vi "LS2A GUI MAIN.vi"() -> ()   [LabVIEW 2015]
panel:
  out "Wired":bool
  out "refnum out":refnum<file>
  out "read buffer":string
  in  "Tab Control":enum32{"Page 1", "Page 2"}(tab)
  out "Bytes Downloaded":dbl
  out "Connection Type":string
  out "Metadata 1":string
  out "Metadata 2":string
  out "Metadata 3":string
  in  "Connect to Unit":bool
  out "System Status":string
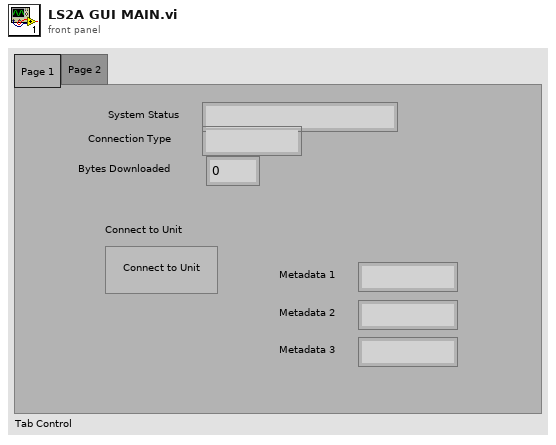
[diagram p1: front panel]
types:
  T1 = enum16{"open", "replace", "create", "open or create", "replace or create", "replace or create with confirmation"}
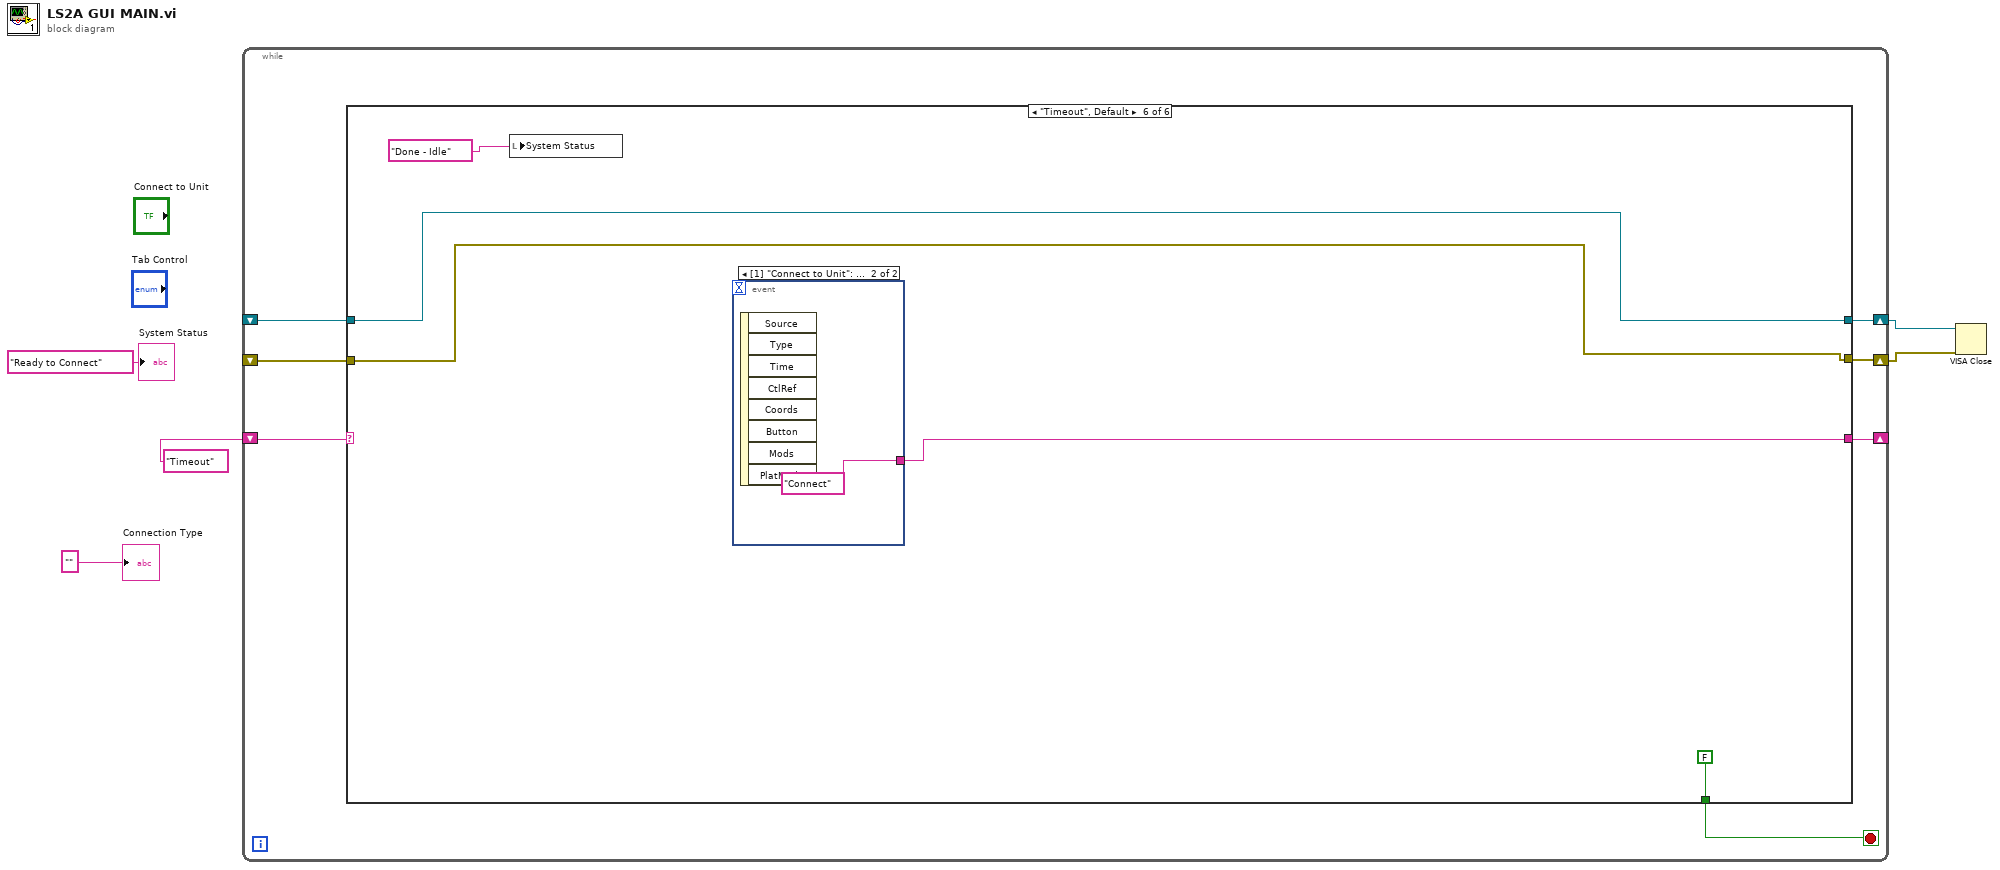
[diagram p0: block diagram]
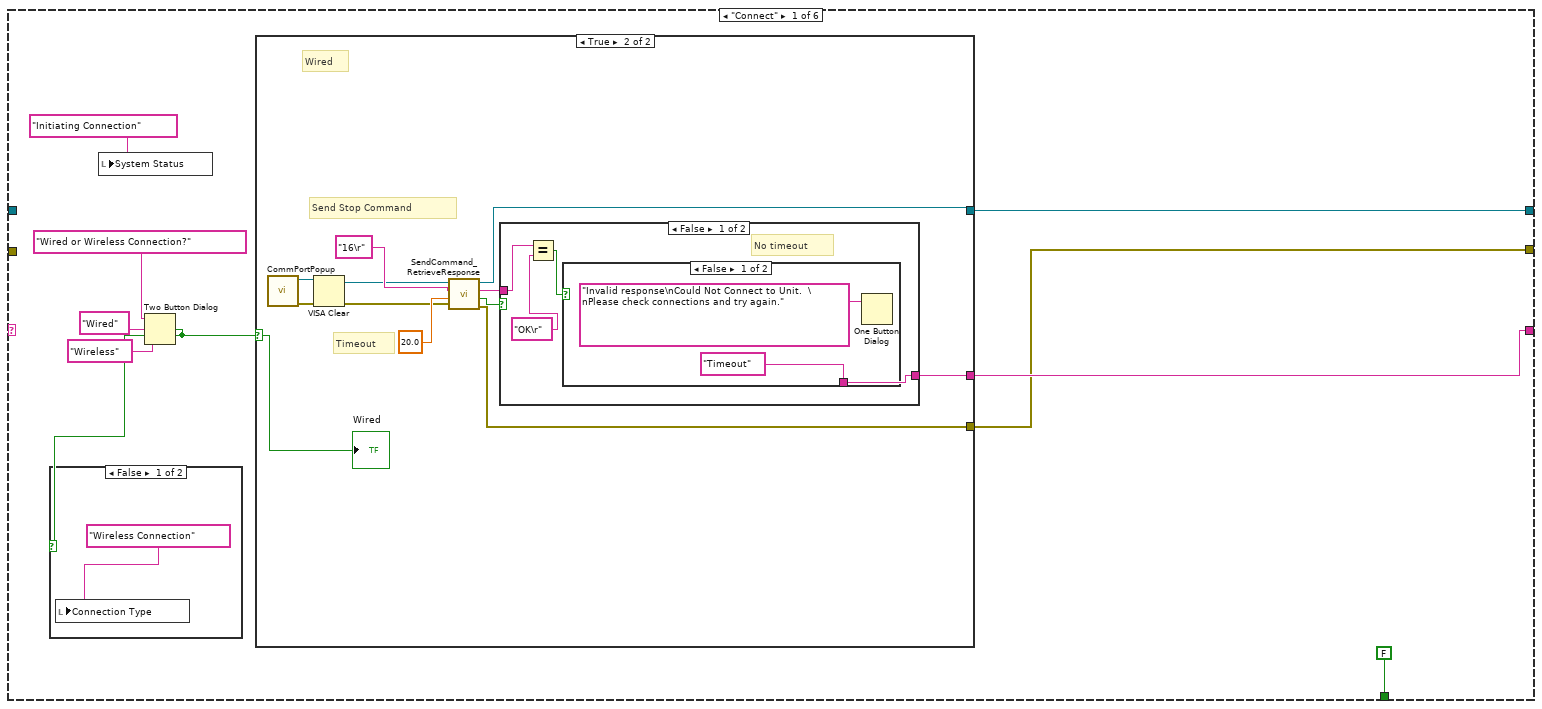
[diagram p2: hidden frame]
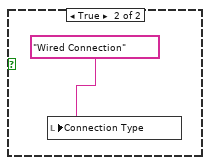
[diagram p3: hidden frame]
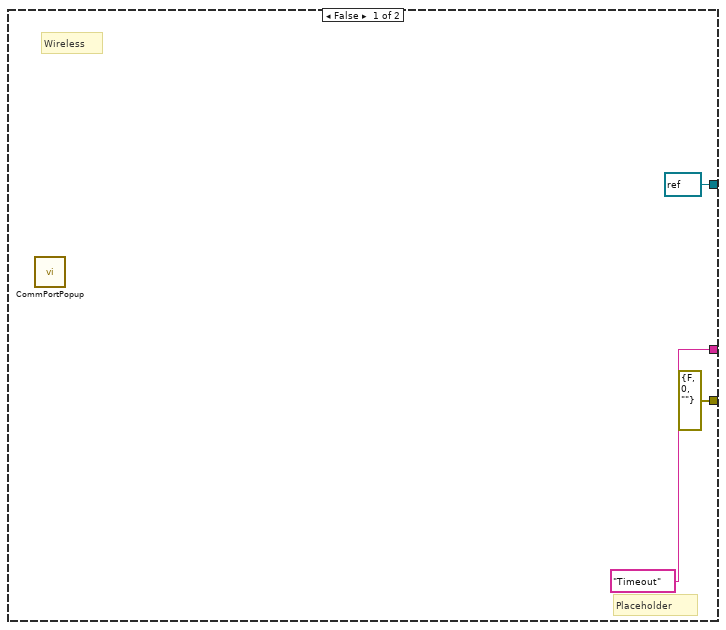
[diagram p4: hidden frame]
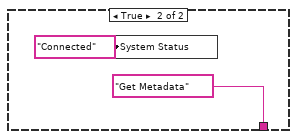
[diagram p5: hidden frame]
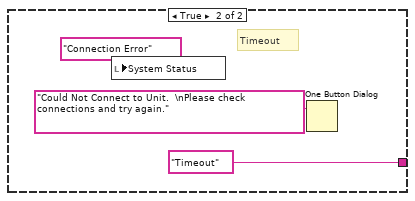
[diagram p6: hidden frame]
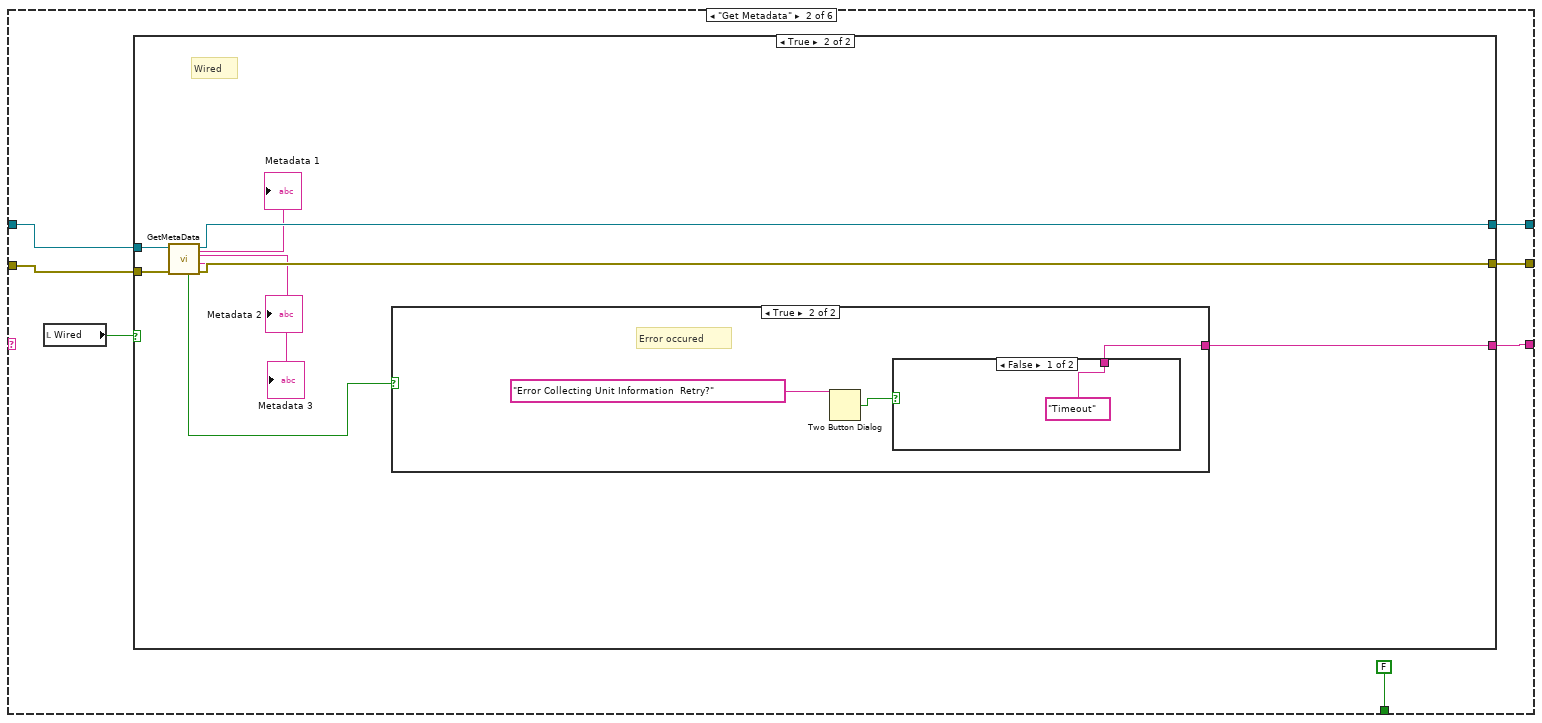
[diagram p7: hidden frame]
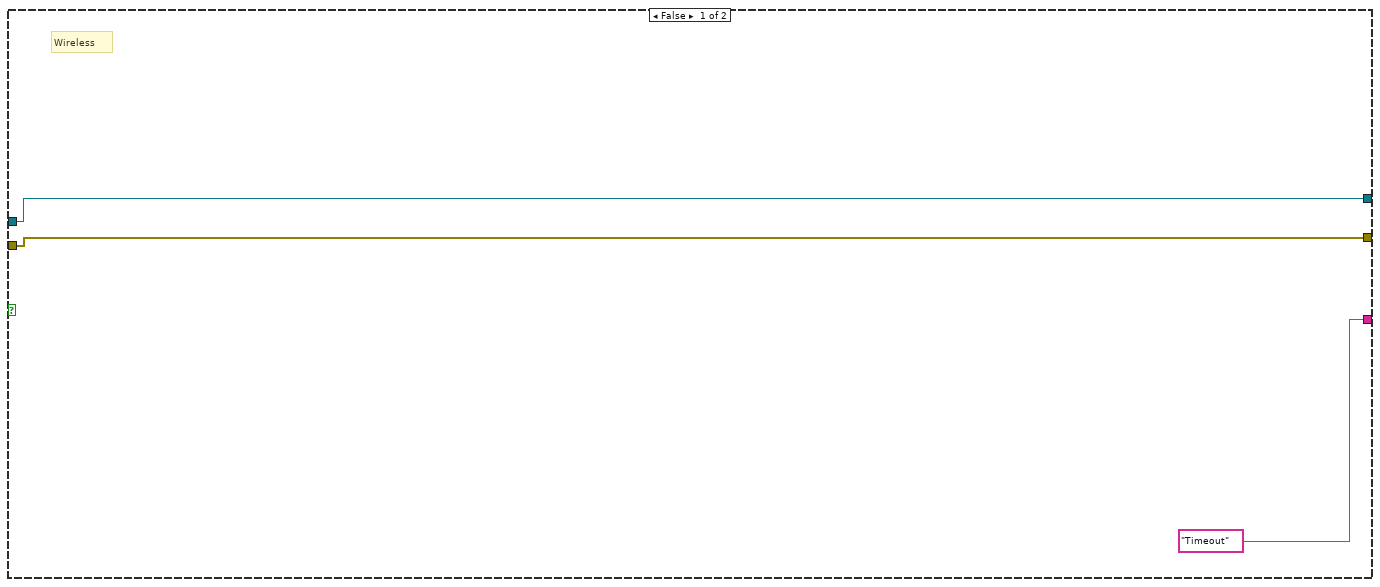
[diagram p8: hidden frame]
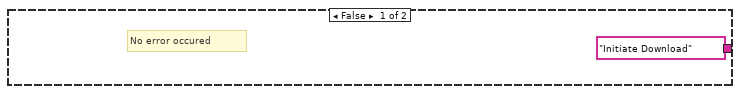
[diagram p9: hidden frame]
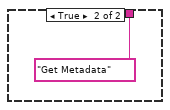
[diagram p10: hidden frame]
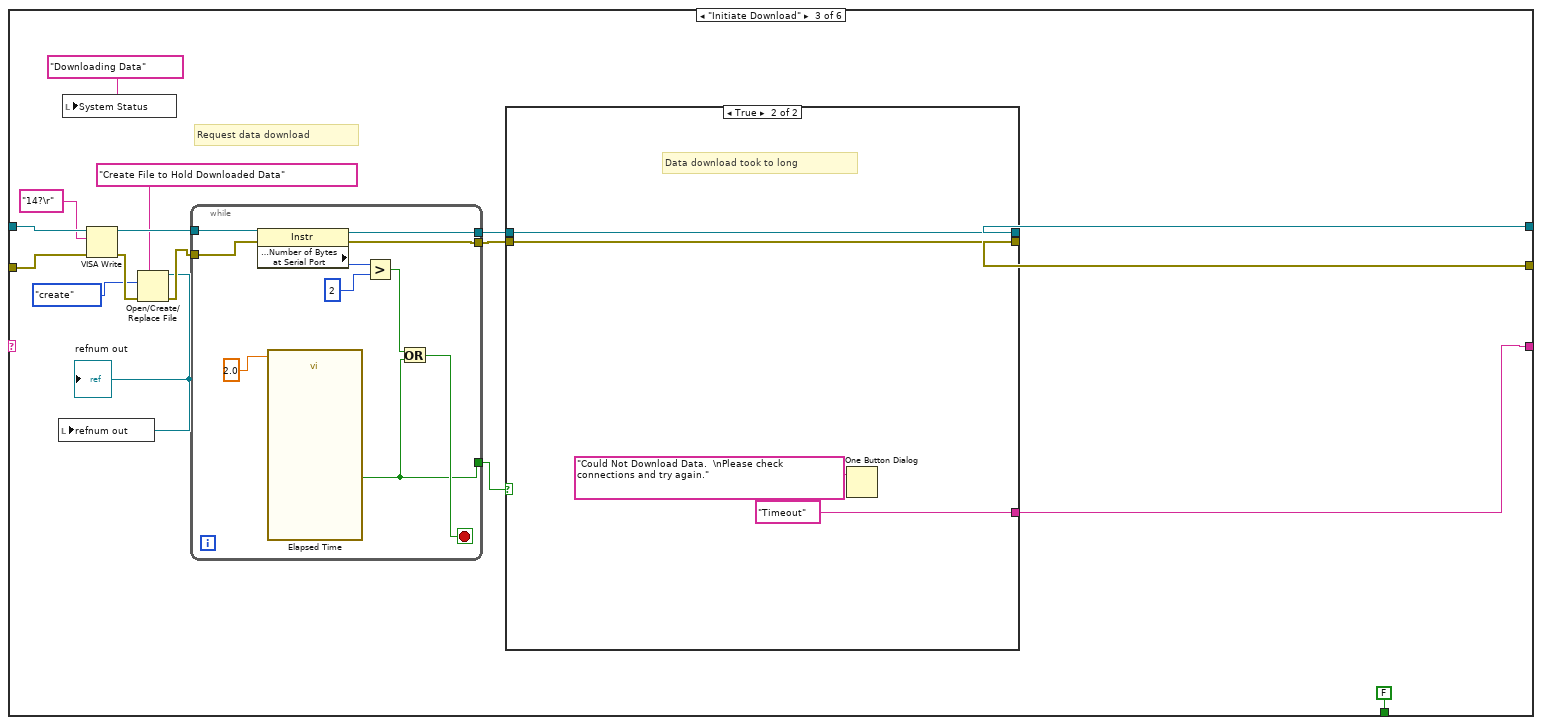
[diagram p11: hidden frame]
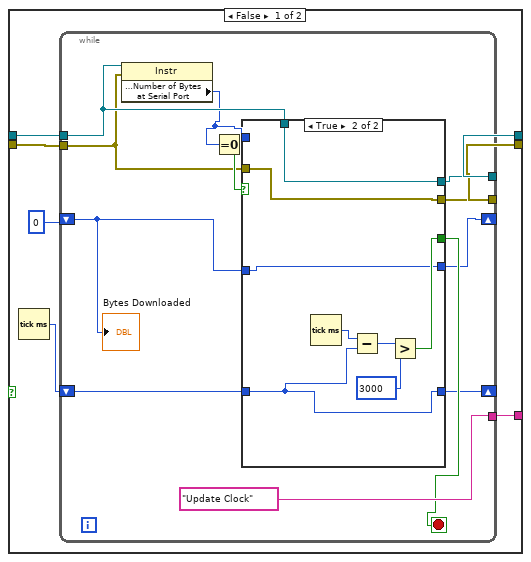
[diagram p12: hidden frame]
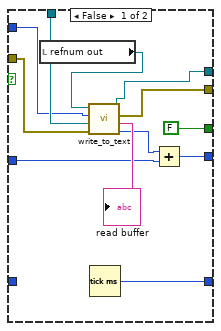
[diagram p13: hidden frame]
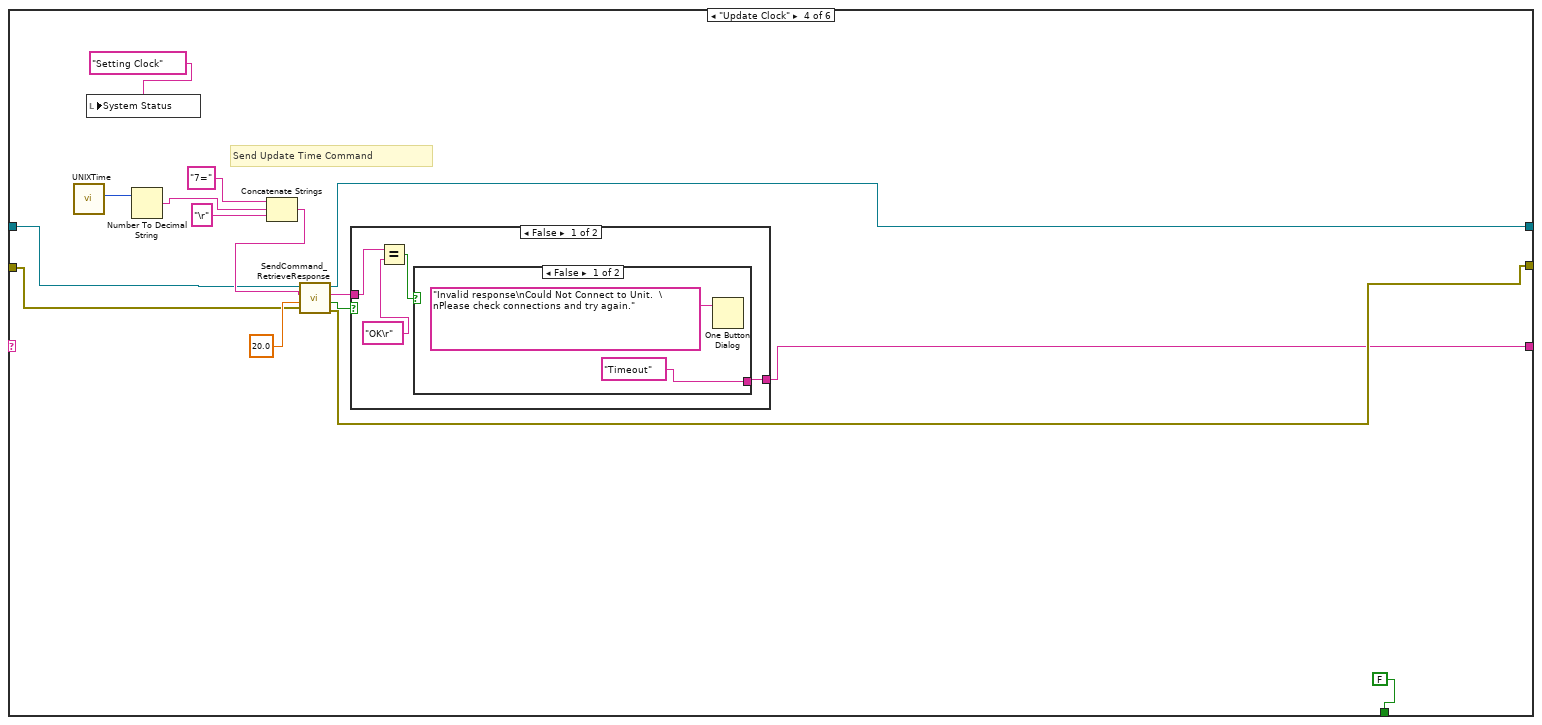
[diagram p14: hidden frame]
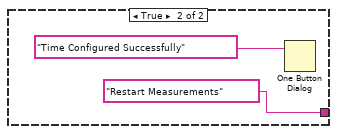
[diagram p15: hidden frame]
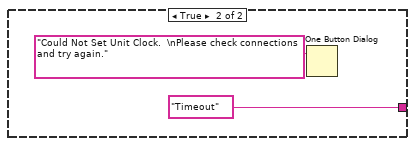
[diagram p16: hidden frame]
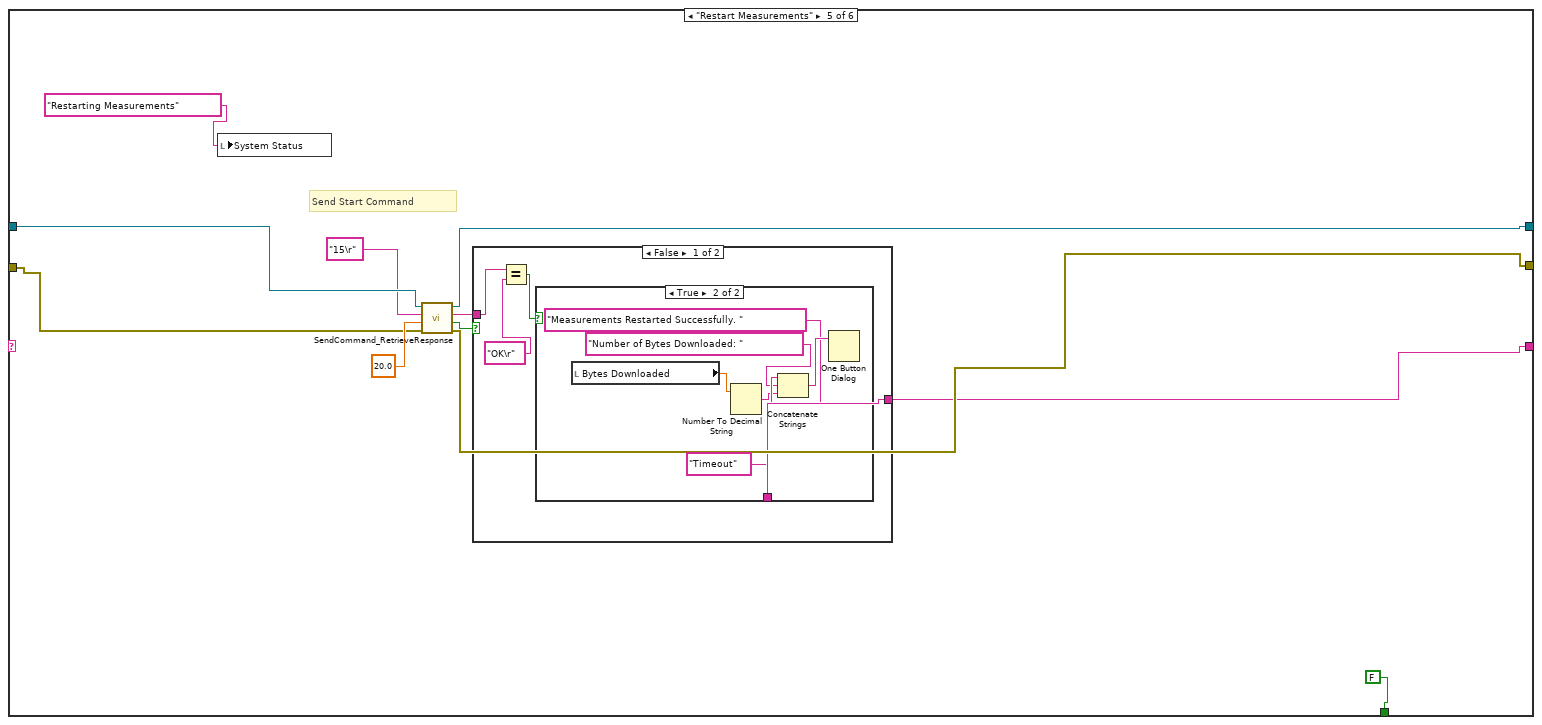
[diagram p17: hidden frame]
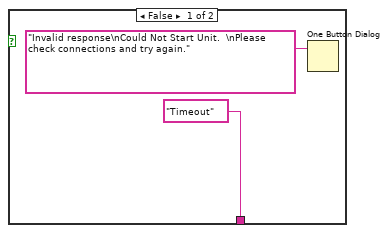
[diagram p18: hidden frame]
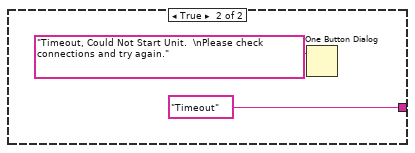
[diagram p19: hidden frame]
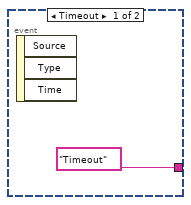
[diagram p20: hidden frame]
diagram:
  n1 = while {
    shift-right: [w11] -> _
    shift-left: "Timeout" -> [w12]
    shift-right: [w9] -> w5
    shift-left: _ -> [w8]
    shift-right: [w10] -> w4
    shift-left: _ -> [w7]
    stop <- w6 stop-if-true
    n2 = case shown="\"Timeout\", Default" w12 {
      tunnel: [w17 w52 w84 w147 w173 w199] -> w11
      tunnel: [w16 w54 w80 w149 w175 w197] -> w10
      tunnel: [w15 w53 w81 w148 w174 w198] -> w9
      tunnel: w8 -> [_ w56 w89 w150 w177 w198]
      tunnel: w7 -> [_ w55 w88 w151 w176 w197]
      tunnel: [FALSE FALSE FALSE FALSE FALSE FALSE] -> w6
      frame "Connect" {
        n3 = local write "System Status"("Initiating Connection" ("System Status")) -> ()
        n4 = Two Button Dialog(message="Wired or Wireless Connection?", 1:"Wireless" ("F button name (\"Cancel\")"), 2:"Wired" ("T button name (\"OK\")")) -> (T button?=w13:bool)
        n5 = case shown="False" w13 {
          frame False {
            n6 = local write "Connection Type"("Wireless Connection" ("String")) -> ()
          }
          frame True {
            n7 = local write "Connection Type"("Wired Connection" ("String")) -> ()
          }
        }
        n8 = case shown="True" w13 {
          selector: w13 -> [_ w27]
          tunnel: ["Timeout" ("System Status") w34] -> w17
          tunnel: [refnum<visa-resource-name> refnum ("VISA Output") w33] -> w15
          tunnel: [errorcluster {"status"=FALSE, "code"=0, "source"=""} ("error out") w32] -> w16
          frame False {
            # "Placeholder"
            # "Wireless"
            n9 = call "CommPortPopup.vi"() -> ()  [unwired: 10 in, 2 out]
          }
          frame True {
            # "Timeout"
            # "Send Stop Command"
            # "Wired"
            n10 = call "CommPortPopup.vi"() -> ("error out"=w31:errorcluster, "VISA resource name out"=w30:refnum<visa-resource-name>)  [unwired: 10 in]
            n11 = VISA Clear(VISA resource name=w30, error in (no error)=w31) -> (VISA resource name out=w28:refnum<visa-resource-name>, error out=w29:errorcluster)
            n12 = call "SendCommand_RetrieveResponse.vi"("error in (no error)"=w29, "Timeout (Seconds)"=20.0, "Input Command"="16\r" ("write buffer"), "VISA Input"=w28) -> ("error out"=w32:errorcluster, "Timeout?"=w36:bool, "System Response"=w35:string, "VISA Output"=w33:refnum<visa-resource-name>)  [unwired: 4 in]
            n13 = case shown="False" w36 {
              tunnel: w35 -> [w41 _]
              tunnel: [w39 "Timeout"] -> w34
              frame False {
                # "No timeout"
                n14 = Equal?(x=w41, y="OK\r") -> (x = y?=w42:bool)
                n15 = case shown="False" w42 {
                  tunnel: ["Timeout" ("System Status") "Get Metadata" ("System Status")] -> w39
                  frame False {
                    n16 = One Button Dialog(message="Invalid response\nCould Not Connect to Unit.  \nPlease check connections and try again.") -> ()  [unwired: 1 in, 1 out]
                  }
                  frame True {
                    n17 = local write "System Status"("Connected" ("System Status")) -> ()
                  }
                }
              }
              frame True {
                # "Timeout"
                n18 = local write "System Status"("Connection Error" ("System Status")) -> ()
                n19 = One Button Dialog(message="Could Not Connect to Unit.  \nPlease check connections and try again.") -> ()  [unwired: 1 in, 1 out]
              }
            }
            "Wired" <- w27
          }
        }
      }
      frame "Get Metadata" {
        n20 = local read "Wired"() -> (w50:bool)
        n21 = case shown="True" w50 {
          tunnel: w56 -> [w59 w68]
          tunnel: w55 -> [w58 w67]
          tunnel: [w58 w66] -> w54
          tunnel: [w59 w65] -> w53
          tunnel: ["Timeout" ("System Status") w60] -> w52
          frame False {
            # "Wireless"
          }
          frame True {
            # "Wired"
            n22 = call "GetMetaData.vi"("error in (no error)"=w67, "VISA Input"=w68) -> ("error out"=w66:errorcluster, "Metadata 3"=→"Metadata 3":string, "Metadata 2"=→"Metadata 2":string, "VISA Output"=w65:refnum<visa-resource-name>, "Error?"=w61:bool, "Metadata 1"=→"Metadata 1":string)  [unwired: 4 in]
            n23 = case shown="True" w61 {
              tunnel: ["Initiate Download" ("System Status") w70] -> w60
              frame False {
                # "No error occured"
              }
              frame True {
                # "Error occured"
                n24 = Two Button Dialog(message="Error Collecting Unit Information  Retry?") -> (T button?=w71:bool)  [unwired: 2 in]
                n25 = case shown="False" w71 {
                  tunnel: ["Timeout" ("System Status") "Get Metadata" ("System Status")] -> w70
                  frame False {
                  }
                  frame True {
                  }
                }
              }
            }
          }
        }
      }
      frame "Initiate Download" {
        # "Request data download"
        n26 = local write "System Status"("Downloading Data" ("System Status")) -> ()
        n27 = VISA Write(VISA resource name=w89, write buffer="14?\r", error in (no error)=w88) -> (VISA resource name out=w86:refnum<visa-resource-name>, error out=w79:errorcluster)  [unwired: 1 out]
        n28 = Open/Create/Replace File(error in=w79, prompt="Create File to Hold Downloaded Data", operation (0:open)=T1."create") -> (refnum out=w76:refnum<file>, error out=w78:errorcluster)  [unwired: 3 in, 1 out]
        "refnum out" <- w76
        n29 = local write "refnum out"(w76) -> ()
        n30 = while {
          tunnel: w86 -> [w144]
          tunnel: w78 -> [w143]
          tunnel: [w135] -> w85
          tunnel: [w137] -> w83
          tunnel: [w136] -> w82
          stop <- w138 stop-if-true
          n31 = property class="Instr"(reference=w144, error in=w143) -> (reference out=w137:refnum<visa-resource-name>, error out=w136:errorcluster, "Serial Settings:Number of Bytes at Serial Port"=w142:u32)
          n32 = call "Elapsed Time"("Time Target (s)"=2.0) -> ("Time has Elapsed"=w135:bool)  [unwired: 11 in, 7 out]
          n33 = Greater?(x=w142, y=u32 2) -> (0:w139:bool)
          n34 = Or(x=w139, y=w135) -> (x .or. y?=w138:bool)
        }
        n35 = case shown="True" w85 {
          tunnel: [w94 "Timeout" ("message")] -> w84
          tunnel: w83 -> [w98 w132]
          tunnel: w82 -> [w97 w131]
          tunnel: [w96 w132] -> w81
          tunnel: [w95 w131] -> w80
          frame False {
            n36 = Tick Count (ms)() -> (millisecond timer value=w93:u32)
            n37 = while {
              tunnel: w98 -> [w109]
              tunnel: w97 -> [w108]
              tunnel: [w106] -> w95
              tunnel: [w105] -> w96
              tunnel: ["Update Clock" ("message")] -> w94
              shift-right: [w102] -> _
              shift-left: w93 -> [w101]
              shift-right: [w100] -> _
              shift-left: 0 -> [w99]
              stop <- w103 stop-if-true
              n38 = property class="Instr"(reference=w109, error in=w108) -> ("Serial Settings:Number of Bytes at Serial Port"=w107:u32)  [unwired: 2 out]
              n39 = Equal To 0?(x=w107) -> (x = 0?=w110:bool)
              n40 = case shown="True" w110 {
                tunnel: w109 -> [w120 w126]
                tunnel: w108 -> [w121 w125]
                tunnel: [FALSE w127] -> w103
                tunnel: w107 -> [w119 _]
                tunnel: [w114 w125] -> w106
                tunnel: [w118 w126] -> w105
                tunnel: [w115 w124] -> w102
                tunnel: w101 -> [_ w124]
                tunnel: [w112 w123] -> w100
                tunnel: w99 -> [w111 w123]
                frame False {
                  n41 = local read "refnum out"() -> (w116:refnum<file>)
                  n42 = call "write_to_text.vi"("error out"=w121, "VISA Output"=w120, "byte count"=w119, "refnum"=w116) -> ("return count"=w113:u32, "read buffer"=→"read buffer":string, "error out 2"=w114:errorcluster, "VISA resource name"=w118:refnum<visa-resource-name>)  [unwired: 4 in]
                  n43 = Tick Count (ms)() -> (millisecond timer value=w115:u32)
                  n44 = Add(x=w113, y=w111) -> (x+y=w112:u32)
                }
                frame True {
                  n45 = Tick Count (ms)() -> (millisecond timer value=w130:u32)
                  n46 = Subtract(x=w130, y=w124) -> (x-y=w129:u32)
                  n47 = Greater?(x=w129, y=u32 3000) -> (0:w127:bool)
                }
              }
              "Bytes Downloaded" <- w99
            }
          }
          frame True {
            # "Data download took to long"
            n48 = One Button Dialog(message="Could Not Download Data.  \nPlease check connections and try again.") -> ()  [unwired: 1 in, 1 out]
          }
        }
      }
      frame "Update Clock" {
        # "Send Update Time Command"
        n49 = call "UNIXTime.vi"() -> ("IntUnixTime 4"=w153:i32)  [unwired: 9 in, 2 out]
        n50 = local write "System Status"("Setting Clock" ("System Status")) -> ()
        n51 = Number To Decimal String(number=w153) -> (decimal integer string=w154:string)  [unwired: 1 in]
        n52 = Concatenate Strings("7=" ("string"), w154, "\r" ("string")) -> (w152:string)
        n53 = call "SendCommand_RetrieveResponse.vi"("error in (no error)"=w151, "Timeout (Seconds)"=20.0, "Input Command"=w152, "VISA Input"=w150) -> ("error out"=w149:errorcluster, "Timeout?"=w158:bool, "System Response"=w157:string, "VISA Output"=w148:refnum<visa-resource-name>)  [unwired: 4 in]
        n54 = case shown="False" w158 {
          tunnel: w157 -> [w162 _]
          tunnel: [w160 "Timeout"] -> w147
          frame False {
            n55 = Equal?(x=w162, y="OK\r") -> (x = y?=w163:bool)
            n56 = case shown="False" w163 {
              tunnel: ["Timeout" ("System Status") "Restart Measurements" ("System Status")] -> w160
              frame False {
                n57 = One Button Dialog(message="Invalid response\nCould Not Connect to Unit.  \nPlease check connections and try again.") -> ()  [unwired: 1 in, 1 out]
              }
              frame True {
                n58 = One Button Dialog(message="Time Configured Successfully") -> ()  [unwired: 1 in, 1 out]
              }
            }
          }
          frame True {
            n59 = One Button Dialog(message="Could Not Set Unit Clock.  \nPlease check connections and try again.") -> ()  [unwired: 1 in, 1 out]
          }
        }
      }
      frame "Restart Measurements" {
        # "Send Start Command"
        n60 = local write "System Status"("Restarting Measurements" ("System Status")) -> ()
        n61 = call "SendCommand_RetrieveResponse.vi"("error in (no error)"=w176, "Timeout (Seconds)"=20.0, "Input Command"="15\r" ("write buffer"), "VISA Input"=w177) -> ("error out"=w175:errorcluster, "Timeout?"=w179:bool, "System Response"=w178:string, "VISA Output"=w174:refnum<visa-resource-name>)  [unwired: 4 in]
        n62 = case shown="False" w179 {
          tunnel: w178 -> [w183 _]
          tunnel: [w181 "Timeout"] -> w173
          frame False {
            n63 = Equal?(x=w183, y="OK\r") -> (x = y?=w184:bool)
            n64 = case shown="True" w184 {
              tunnel: ["Timeout" ("System Status") "Timeout" ("System Status")] -> w181
              frame False {
                n65 = One Button Dialog(message="Invalid response\nCould Not Start Unit.  \nPlease check connections and try again.") -> ()  [unwired: 1 in, 1 out]
              }
              frame True {
                n66 = local read "Bytes Downloaded"() -> (w191:dbl)
                n67 = Number To Decimal String(number=w191) -> (decimal integer string=w187:string)  [unwired: 1 in]
                n68 = Concatenate Strings("Measurements Restarted Successfully. " ("message"), "Number of Bytes Downloaded: " ("message"), w187) -> (w190:string)
                n69 = One Button Dialog(message=w190) -> ()  [unwired: 1 in, 1 out]
              }
            }
          }
          frame True {
            n70 = One Button Dialog(message="Timeout, Could Not Start Unit.  \nPlease check connections and try again.") -> ()  [unwired: 1 in, 1 out]
          }
        }
      }
      frame "Timeout", Default {
        n71 = local write "System Status"("Done - Idle" ("System Status")) -> ()
        n72 = event shown="[1] \"Connect to Unit\": Mouse Up" {
          selector: _ -> [_ _]
          dyn-events: _ -> [_ _]
          timeout: _ -> [_ _]
          tunnel: ["Timeout" "Connect"] -> w199
          event Timeout {
            n73 = event-data() -> ()  [unwired: 1 in, 3 out]
          }
          event "Connect to Unit": Mouse Up {
            n74 = event-data() -> ()  [unwired: 1 in, 8 out]
          }
        }
      }
    }
  }
  n75 = VISA Close(VISA resource name=w5, error in (no error)=w4) -> ()  [unwired: 1 out]
  "System Status" <- "Ready to Connect" ("System Status")
  "Connection Type" <- "" ("String")
